vi "F-FormularFilterProcess.vi"() -> ()   [LabVIEW 2014]
doc: "Use this template to build a VI to use as a subVI."
uses:
  <vilib>/vision/NI_Vision_Development_Module.lvlib
panel:
  in  "v0":i16=60
  in  "u0":i16=128
  in  "D1":u16=40
  in  "D0":u16=20
  in  "N-Order":u8(slide)=2 scale=0.0..10.0
  in  "Filter":T1(ring)=enum."GHPF"
  out "|F(u,v)H(u,v)|":T2(plugin-control)
  out "g(x,y)":T2(plugin-control)
  out "IF(u,v)I":T2(plugin-control)
  out "f(x,y)":T2(plugin-control)
  # "1) low/high pass filter controlled by D0;\n2) Band pass/reject controlled by D0(low cut) and D1(high cut);\n3) Notch Filter controlled by (+/-u0,+/-v0) and D0;"
  # ":: MVi Framework V1.0 ::\nAuthor:Gaoke Yang\nEmail: gaoke.yang@yahoo.com\nWeb: www.mvicontrol.com\nCopyright (C) 2015, MVI Technologies All Rights Reserved"
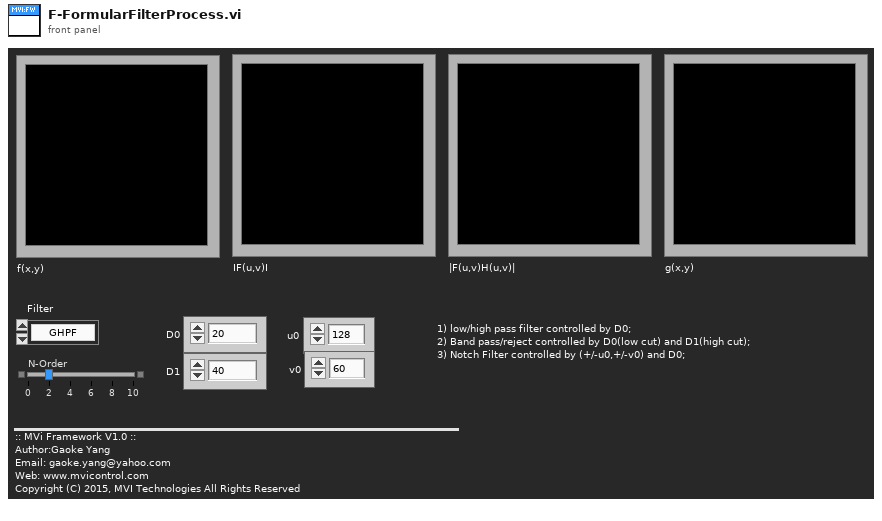
[diagram p1: front panel]
types:
  T1 = enum16{"ILPF", "IHPF", "IBPF", "IBRF", "BLPF", "BHPF", "BBPF", "BBRF", "ELPF", "EHPF", "EBPF", "EBRF", "GLPF", "GHPF", "GBPF", "GBRF"}
  T2 = typedef "IMAQ Image.ctl" = refnum<image>
  T3 = typedef "Image Type" = u32
  T4 = cluster{"D0":u16, "D1":u16, "u0":i16, "v0":i16, "N-Order":u8}
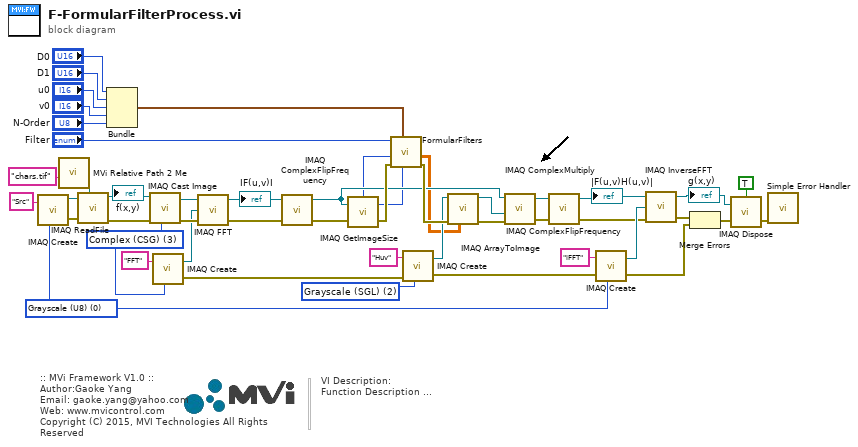
[diagram p0: block diagram]
diagram:
  w14 = T3 2 items=["Grayscale (U8)", "Grayscale (I16)", "Grayscale (SGL)", "Complex (CSG)", "RGB (U32)", "HSL (U32)", "RGB (U64)", "Grayscale (U16)"] ("Image Type")
  w7 = T3 0 items=["Grayscale (U8)", "Grayscale (I16)", "Grayscale (SGL)", "Complex (CSG)", "RGB (U32)", "HSL (U32)", "RGB (U64)", "Grayscale (U16)"] ("Image Type")
  w12 = T3 3 items=["Grayscale (U8)", "Grayscale (I16)", "Grayscale (SGL)", "Complex (CSG)", "RGB (U32)", "HSL (U32)", "RGB (U64)", "Grayscale (U16)"] ("Image Type")
  # "VI Description:\nFunction Description ..."
  # ":: MVi Framework V1.0 ::\nAuthor:Gaoke Yang\nEmail: gaoke.yang@yahoo.com\nWeb: www.mvicontrol.com\nCopyright (C) 2015, MVI Technologies All Rights Reserved"
  n1 = call "IMAQ Create"("Image Name"="Src" ("name or relative path"), "Image Type"=w7) -> ("New Image"=w45:T2, "error out"=w44:errorcluster)  [unwired: 2 in, 1 out]
  n2 = call "MVi Relative Path 2 Me.vi"("Relative Path"="chars.tif" ("name or relative path")) -> ("Appended Dir"=w41:path)  [unwired: 5 in, 1 out]
  n3 = call "IMAQ ReadFile"("File Path"=w41, "error in (no error)"=w44, "Image"=w45) -> ("error out"=w38:errorcluster, "Image Out"=w37:T2)  [unwired: 4 in, 3 out]
  "f(x,y)" <- w37
  n4 = Bundle("D0"="D0", "D1"="D1", "u0"="u0", "v0"="v0", "N-Order"="N-Order") -> (w1:T4)  [unwired: 1 in]
  n5 = call "IMAQ Cast Image"("Image Type"=w12, "error in (no error)"=w38, "Image Src"=w37) -> ("error out"=w40:errorcluster, "Image Dst Out"=w36:T2)  [unwired: 7 in]
  n6 = call "IMAQ Create"("Image Name"="FFT" ("name or relative path"), "Image Type"=w12) -> ("New Image"=w35:T2, "error out"=w33:errorcluster)  [unwired: 2 in, 1 out]
  n7 = call "IMAQ FFT"("error in (no error)"=w40, "Image Dst"=w35, "Image Src"=w36) -> ("error out"=w30:errorcluster, "Image Dst Out"=w29:T2)  [unwired: 1 in]
  "IF(u,v)I" <- w29
  n8 = call "IMAQ ComplexFlipFrequency"("error in (no error)"=w30, "Image Src"=w29) -> ("error out"=w24:errorcluster, "Image Dst Out"=w18:T2)  [unwired: 2 in]
  n9 = call "IMAQ GetImageSize"("Image"=w18, "error in (no error)"=w24) -> ("Y Resolution"=w11:i32, "X Resolution"=w10:i32, "error out"=w23:errorcluster)  [unwired: 2 in]
  n10 = call "FormularFilters.vi"("ImgY"=w11, "FilterParam"=w1, "EorIn"=w23, "ImgX"=w10, "Filter"="Filter") -> ("ErrOut"=w22:errorcluster, "H(u,v)"=w8:dbl[][])  [unwired: 5 in]
  n11 = call "IMAQ Create"("Image Name"="Huv" ("name or relative path"), "Image Type"=w14, "error in (no error)"=w33) -> ("New Image"=w15:T2, "error out"=w16:errorcluster)  [unwired: 1 in, 1 out]
  n12 = call "IMAQ ArrayToImage"("Image Pixels (Float)"=w8, "error in (no error)"=w22, "Image"=w15) -> ("error out"=w17:errorcluster, "Image Out"=w13:T2)  [unwired: 7 in]
  n13 = call "IMAQ ComplexMultiply"("Image Src A"=w18, "Image Src B"=w13, "error in (no error)"=w17) -> ("Image Dst Out"=w27:T2, "error out"=w28:errorcluster)  [unwired: 4 in]
  n14 = call "IMAQ ComplexFlipFrequency"("error in (no error)"=w28, "Image Src"=w27) -> ("error out"=w26:errorcluster, "Image Dst Out"=w25:T2)  [unwired: 2 in]
  "|F(u,v)H(u,v)|" <- w25
  n15 = call "IMAQ Create"("Image Name"="iFFT" ("name or relative path"), "Image Type"=w7, "error in (no error)"=w16) -> ("New Image"=w31:T2, "error out"=w19:errorcluster)  [unwired: 1 in, 1 out]
  n16 = call "IMAQ InverseFFT"("error in (no error)"=w26, "Image Dst"=w31, "Image Src"=w25) -> ("error out"=w21:errorcluster, "Image Dst Out"=w20:T2)  [unwired: 1 in]
  "g(x,y)" <- w20
  n17 = Merge Errors(w21, w19) -> (w39:errorcluster)
  n18 = call "IMAQ Dispose"("All Images? (No)"=TRUE, "Image"=w20, "error in (no error)"=w39) -> ("error out"=w46:errorcluster)  [unwired: 3 out]
  n19 = call <vilib>:"Simple Error Handler.vi"("error in (no error)"=w46) -> ()  [unwired: 1 in, 8 out]
